vi "Drive.vi"(8 "error in (no error)":errorcluster, 9 "Turn":sgl, 10 "Drive":sgl, 11 "Rover in":refnum<class "Rover.lvclass">) -> (0 "error out":errorcluster, 3 "Rover out":refnum<class "Rover.lvclass">)   [LabVIEW 2020, in "Rover.lvlib" / "Rover.lvclass"]
uses:
  Rover.lvclass
  I2C Register.ctl
  Flags.ctl
  Rover.lvclass/Rover.ctl
  <vilib>/MakerHub/LINX/Private/Local IO/LinxI2cWrite.vi
  <vilib>/MakerHub/LINX/Public/Utilities/Check Channel.vi
  <vilib>/MakerHub/LINX/Private/Local IO/Handle Errors.vi
  <vilib>/MakerHub/LINX/Private/Utilties/Generate Error.vi
  <vilib>/MakerHub/LINX/LMH-LINX.lvlib
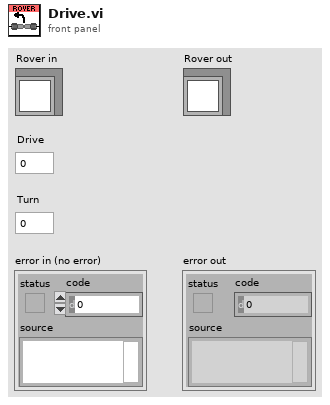
[diagram p1: front panel]
types:
  T1 = typedef "Rover.lvlib/Rover.lvclass/Flags.ctl" = cluster{"Reset":bool, "Run":bool, "Brake":bool, "Coast":bool, "Unused 1":bool, "Unused 2":bool, "Unused 3":bool, "Unused 4":bool}
  T2 = typedef "Rover.lvlib/Rover.lvclass/I2C Register.ctl" = enum8{"encA", "encB", "ticksPerUnit", "width", "flags", "velP", "velI", "velD", "velMin", "velMax", "poseX", "poseY", "poseA", "cmdDrive", "cmdTurn", "velocity", "turn", "velL", "velR", "run", "outL", "outR", "outDeadband"}
  T3 = typedef "LMH-LINX.lvlib/LINX Ref.ctl" = cluster{"IO":T4, "Interface":T5, "LINX Device Config":T6}
  T4 = typedef "LMH-LINX.lvlib/Platform.ctl" = enum16{"Remote", "Local"}
  T5 = typedef "LMH-LINX.lvlib/Interface.ctl" = enum16{"Serial", "TCP"}
  T6 = typedef "LMH-LINX.lvlib/Device.lvlib/LINX Device Config.ctl" = cluster{"Interface":T5, "COM Port":refnum<visa-resource-name>, "TCP Configuration":T7, "Device Family":u8, "Device ID":u8, "Device Name":string, "TCP Ref":refnum<k5>, "Channels":T8}
  T7 = typedef "LMH-LINX.lvlib/Device.lvlib/TCP Config.ctl" = cluster{"IP Address":string, "Port":u16}
  T8 = typedef "LMH-LINX.lvlib/Channels.ctl" = cluster{"DI":u8[], "DO":u8[], "AI":u8[], "AO":u8[], "PWM":u8[], "QE":u8[], "UART":u8[], "I2C 2":u8[], "SPI":u8[], "CAN":u8[], "Servo":u8[], "AI Ref (V)":dbl, "AI Resolution (Bits)":u8, "AO Ref (V)":dbl, "AO Resolution (Bits)":u8}
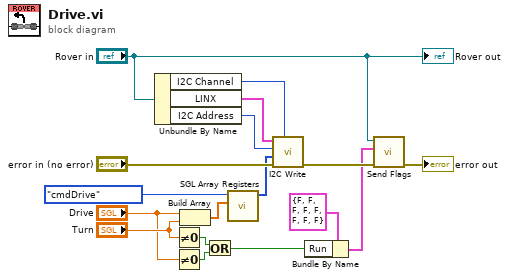
[diagram p0: block diagram]
diagram:
  n1 = Unbundle By Name("Rover in") -> ("I2C Channel"=w16:u8, "LINX"=w14:T3, "I2C Address"=w15:u8)
  n2 = Not Equal To 0?(x="Turn") -> (x != 0?=w3:bool)
  n3 = Not Equal To 0?(x="Drive") -> (x != 0?=w2:bool)
  n4 = Build Array("Drive", "Turn") -> (w12:sgl[])
  n5 = Or(x=w3, y=w2) -> (x .or. y?=w1:bool)
  n6 = call "SGL Array Registers.vi"("SGL Array"=w12, "I2C Register"=I2C_Register."cmdDrive" ("Register")) -> ("Data"=w11:u8[])  [unwired: 9 in]
  n7 = call <vilib>:"I2C Write.vi"("I2C Channel"=w16, "Error In"="error in (no error)", "Data"=w11, "I2C Slave Address (0)"=w15, "LINX Resource"=w14) -> ("Error Out"=w10:errorcluster)  [unwired: 5 in, 1 out]
  n8 = Bundle By Name(cluster=T1 {"Reset"=FALSE, "Run"=FALSE, "Brake"=FALSE, "Coast"=FALSE, "Unused 1"=FALSE, "Unused 2"=FALSE, "Unused 3"=FALSE, "Unused 4"=FALSE} ("Flags"), "Run"=w1) -> (w6:T1)
  n9 = call "Send Flags.vi"("error in (no error)"=w10, "Flags"=w6, "Rover in"="Rover in") -> ("error out"=→"error out":errorcluster)  [unwired: 7 in, 1 out]
  "Rover out" <- "Rover in"
